vi "Write Scan info txt and ini file.vi"(0 "Scan/NoScan":T2, 2 "Scan setup":T1={"Scan Start"=1.0, "Scan End"=10.0, "Scan Step Size"=1.0, "# Shots Each Step"=10, "single direction?"=TRUE} {"Scan Start" format="%#.9p"; "Scan End" format="%#.9p"; "Scan Step Size" format="%#.9p"}, 5 "Scan Info":string, 7 "ScanInfo file path":path, 9 "Scan Number":i32, 11 "Scans Path":path, 12 "Active Variable":string, 13 "Active Device":string, 14 "error in":errorcluster) -> (15 "error out":errorcluster)   [LabVIEW 2018]
doc: "This vi write scan info in text and in configuration file."
uses:
  Scan Tab Enum.ctl
  scan parameters.ctl
  <vilib>/Utility/config.llb/Write Key (String).vi
  <vilib>/Utility/config.llb/Write Key (Double).vi
  <vilib>/Utility/config.llb/Write Key (U32).vi
  <vilib>/Utility/config.llb/NI_LVConfig.lvlib
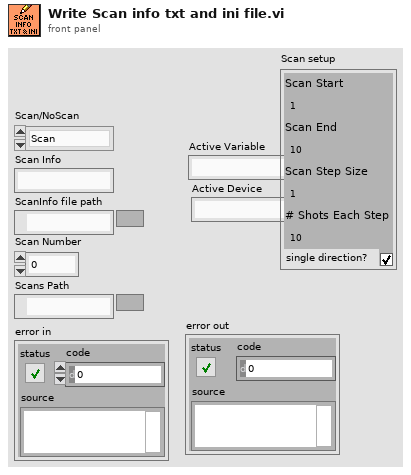
[diagram p1: front panel]
types:
  T1 = typedef "scan parameters.ctl" = cluster{"Scan Start":dbl, "Scan End":dbl, "Scan Step Size":dbl, "# Shots Each Step":u32, "single direction?":bool}
  T2 = typedef "Scan Tab Enum.ctl" = enum32{"Scan", "File Scan", "NoScan", "Saved Scans"}
  T3 = typedef "NI_LVConfig.lvlib/Config Data RefNum.ctl" = refnum<k1>
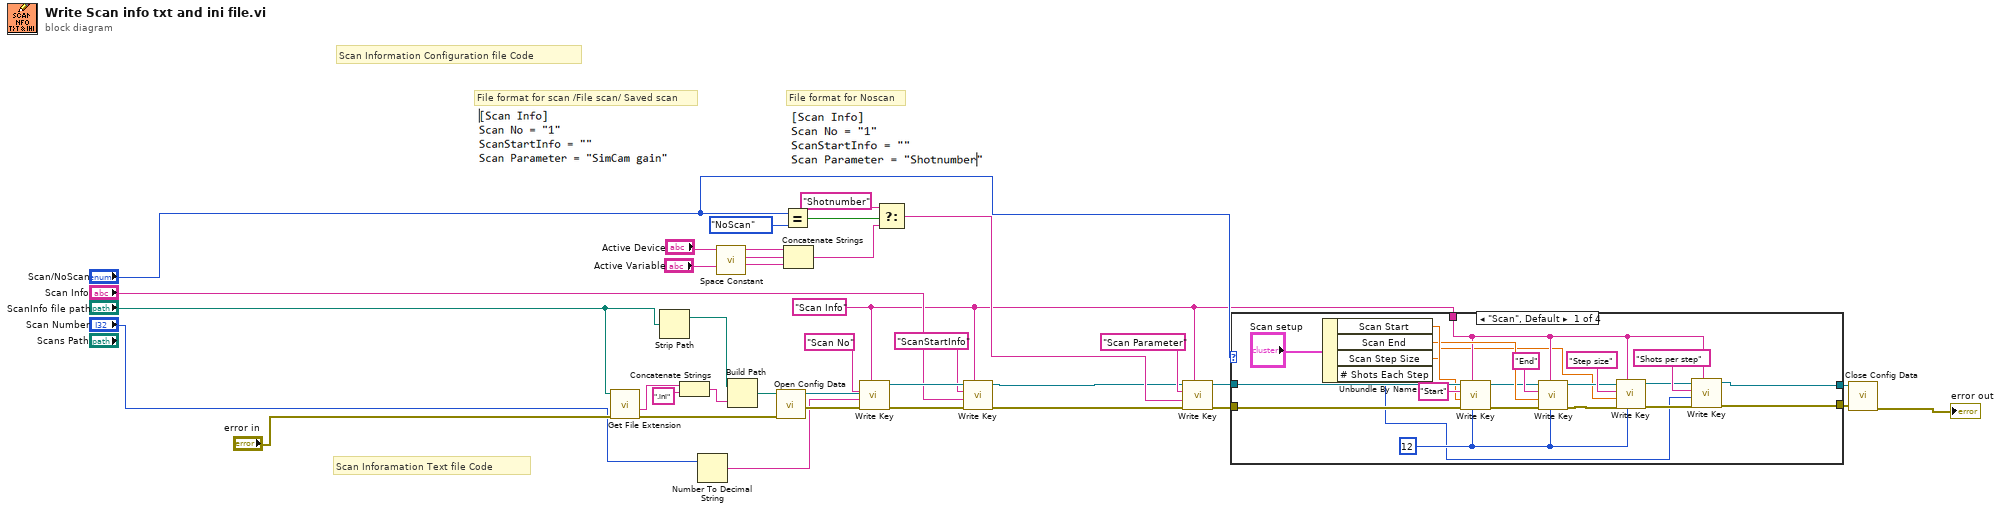
[diagram p0: block diagram]
diagram:
  w6 = "Scan Info" ("section")
  # "Scan Inforamation Text file Code"
  # "Scan Information Configuration file Code"
  # "File format for Noscan"
  # "File format for scan /File scan/ Saved scan"
  n1 = call <vilib>:"Get File Extension.vi"("error in (no error)"="error in", "file"="ScanInfo file path") -> ("error out"=w25:errorcluster, "filename without extension"=w21:string)  [unwired: 5 in, 3 out]
  n2 = Strip Path(path="ScanInfo file path") -> (stripped path=w22:path)  [unwired: 1 out]
  n3 = Concatenate Strings(w21, ".ini" ("string")) -> (w23:string)
  n4 = Number To Decimal String(number="Scan Number") -> (decimal integer string=w2:string)  [unwired: 1 in]
  n5 = call <vilib>:"Space Constant.vi"() -> ("String"=w19:string)
  n6 = Build Path(base path=w22, name or relative path=w23) -> (appended path=w24:path)
  n7 = call <vilib>:"Open Config Data.vi"("error in (no error)"=w25, "configuration file path"=w24) -> ("error out"=w18:errorcluster, "refnum"=w28:T3)  [unwired: 7 in, 1 out]
  n8 = Equal?(x="Scan/NoScan", y=Scan_Tab_Enum."NoScan" ("Scan/NoScan")) -> (x = y?=w32:bool)
  n9 = Concatenate Strings("Active Device", w19, "Active Variable") -> (w34:string)
  n10 = call-poly <vilib>:"Write Key.vi"("section"=w6, "error in (no error)"=w18, "value"=w2, "key"="Scan No", "refnum"=w28) -> ("error out"=w17:errorcluster, "refnum out"=w29:T3)  [unwired: 4 in, 1 out]
  n11 = Select(t="Shotnumber" ("key"), s=w32, f=w34) -> (s? t:f=w35:string)
  n12 = call-poly <vilib>:"Write Key.vi"("section"=w6, "error in (no error)"=w17, "value"="Scan Info", "key"="ScanStartInfo", "refnum"=w29) -> ("error out"=w4:errorcluster, "refnum out"=w5:T3)  [unwired: 4 in, 1 out]
  n13 = call-poly <vilib>:"Write Key.vi"("section"=w6, "error in (no error)"=w4, "value"=w35, "key"="Scan Parameter", "refnum"=w5) -> ("error out"=w9:errorcluster, "refnum out"=w10:T3)  [unwired: 4 in, 1 out]
  n14 = case shown="\"Scan\", Default" "Scan/NoScan" {
    tunnel: w10 -> [w56 w58 w60 w62]
    tunnel: w6 -> [w41 _ _ _]
    tunnel: w9 -> [w52 w57 w59 w61]
    tunnel: [w40 w58 w60 w62] -> w8
    tunnel: [w39 w57 w59 w61] -> w7
    frame "Scan", Default {
      w38 = i16 12 ("precision (6)")
      n15 = Unbundle By Name("Scan setup") -> ("Scan Start"=w53:dbl, "Scan End"=w51:dbl, "Scan Step Size"=w37:dbl, "# Shots Each Step"=w36:u32)
      n16 = call-poly <vilib>:"Write Key.vi"("precision (6)"=w38, "section"=w41, "error in (no error)"=w52, "value"=w53, "key"="Start", "refnum"=w56) -> ("error out"=w48:errorcluster, "refnum out"=w49:T3)  [unwired: 3 in, 1 out]
      n17 = call-poly <vilib>:"Write Key.vi"("precision (6)"=w38, "section"=w41, "error in (no error)"=w48, "value"=w51, "key"="End", "refnum"=w49) -> ("error out"=w46:errorcluster, "refnum out"=w45:T3)  [unwired: 3 in, 1 out]
      n18 = call-poly <vilib>:"Write Key.vi"("precision (6)"=w38, "section"=w41, "error in (no error)"=w46, "value"=w37, "key"="Step size", "refnum"=w45) -> ("error out"=w43:errorcluster, "refnum out"=w42:T3)  [unwired: 3 in, 1 out]
      n19 = call-poly <vilib>:"Write Key.vi"("section"=w41, "error in (no error)"=w43, "value"=w36, "key"="Shots per step", "refnum"=w42) -> ("error out"=w39:errorcluster, "refnum out"=w40:T3)  [unwired: 4 in, 1 out]
    }
    frame "File Scan" {
    }
    frame "NoScan" {
    }
    frame "Saved Scans" {
    }
  }
  n20 = call <vilib>:"Close Config Data.vi"("error in (no error)"=w7, "refnum"=w8) -> ("error out"=→"error out":errorcluster)  [unwired: 8 in, 1 out]
